vi "Server Sim.vi"() -> ()   [LabVIEW 2015]
uses:
  Type/TCP Packet Info.ctl
  Type/_RT Command.ctl
panel:
  in  "Stop Button":bool
  out "State":i32
  out "Response":string
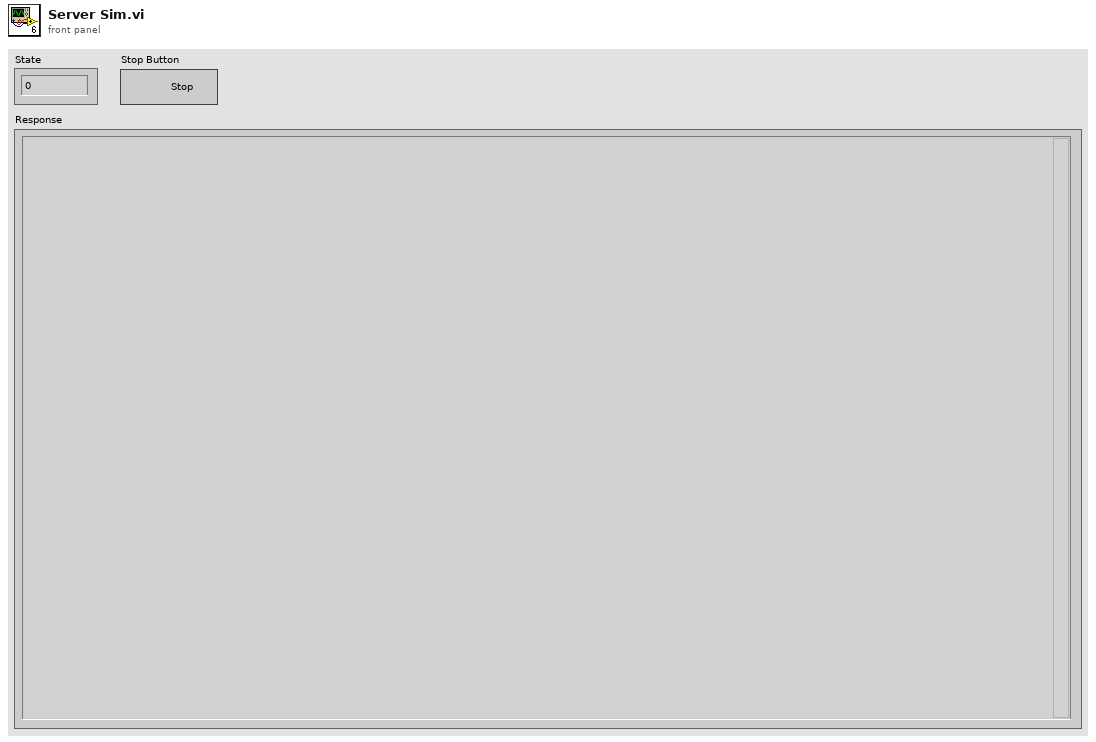
[diagram p1: front panel]
types:
  T1 = typedef "_RT Command.ctl" = enum16{"xml Start Run", "xml Start Actual Run", "xml Stop Run", "xml Runtime Update", "xml Get Status", "xml Get Table", "xml Set Table", "xml Get Configuration", "xml System Status", "xml Set LC Input Logic", "xml Get Data", "xml Get Info", "Start", "StartActualRun", "Stop", "Runtime Update", "Get Data", "Get Info", "Get Status", "Get Param", "Get Config", "Get Table", "Read ADC", "Set Oscillator", "Update Config", "Update Table", "Set All Pol", "Set Pol and DC", "Set Max Mass", "Toggle RP", "Toggle EL", "Set PIC", "Initialize Turbo", "Send Turbo Comm", "Close Turbo", "P1", "P2", "P3", "Send Serial", "Set LC Out", "Get LC In", "Read VAC", "Test Table", "Toggle Power", "Get Startup", "Set Startup", "Get ADC Table", "Set ADC Table", "Get Brief Status", "Get Detail Status", "Auxiliary Update", "Set CC Logics", "Set CC Input Logics", "Ignore Error", "invalid"}
  T2 = typedef "TCP Packet Info.ctl" = cluster{"Packet Signature":string, "Sequence Number":i32, "Command":T1, "Data Message Size":u32, "Data Message Size":string, "Data Message":string, "Error Message Size":u32, "Error Message Size":string, "Error Message":string, "Checksum":u32, "Error Message":errorcluster, "Command ID":string}
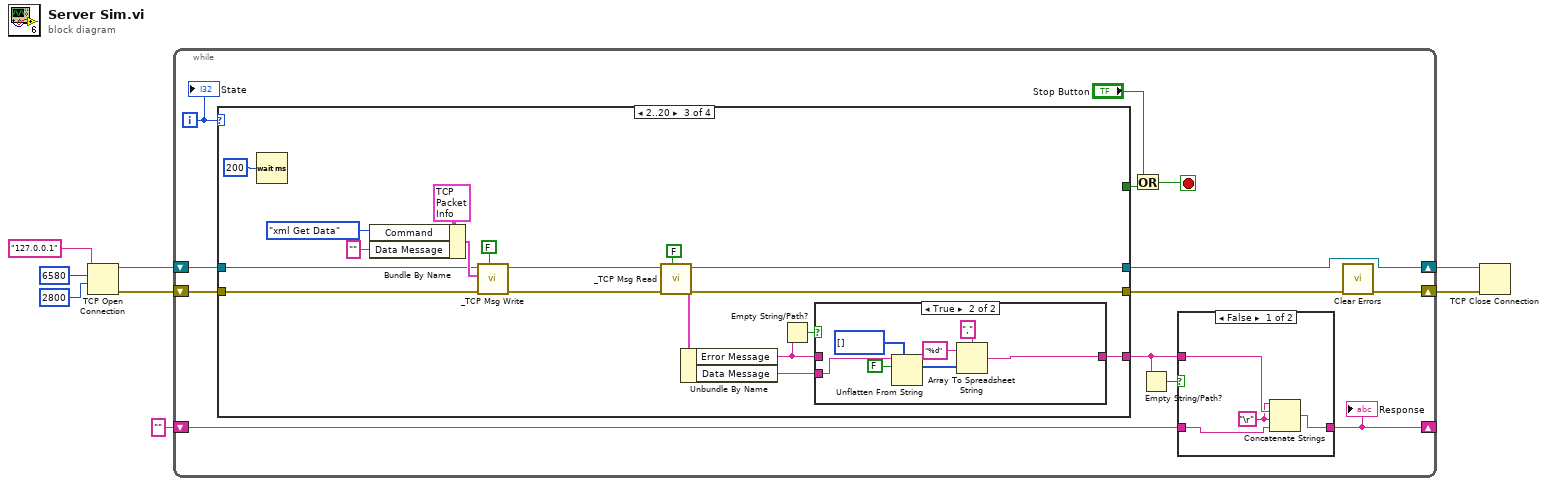
[diagram p0: block diagram]
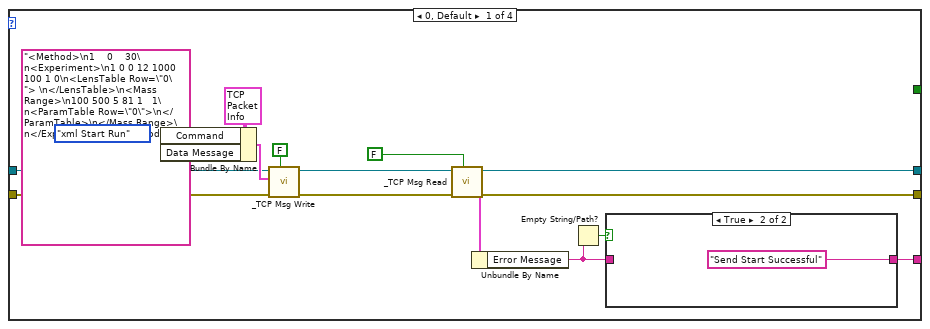
[diagram p3: hidden frame]
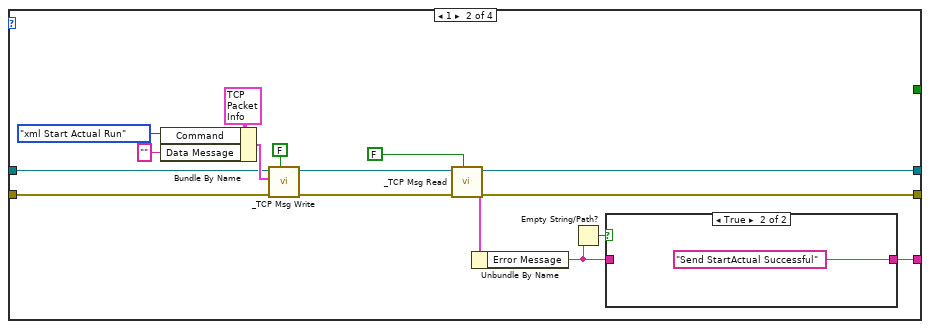
[diagram p5: hidden frame]
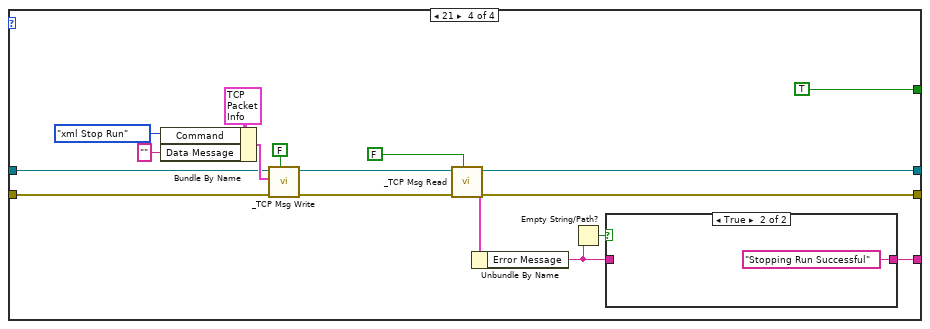
[diagram p8: hidden frame]
diagram:
  n1 = TCP Open Connection(address="127.0.0.1", remote port or service name=u16 6580 ("remote port"), timeout ms (60000)=2800) -> (connection ID=w5:refnum<k5>, error out=w4:errorcluster)  [unwired: 1 in, 1 out]
  n2 = while {
    shift-right: [w19] -> w3
    shift-left: w4 -> [w21]
    shift-right: [w16] -> w2
    shift-left: w5 -> [w20]
    shift-right: [w14] -> _
    shift-left: "" ("Data Message") -> [w15]
    i -> [w18]
    stop <- w10 stop-if-true
    n3 = case shown="2..20" w18 {
      tunnel: w21 -> [w38 w56 w76 w101]
      tunnel: w20 -> [w37 w55 w75 w100]
      tunnel: [w31 w49 w69 w94] -> w17
      tunnel: [w32 w50 w70 w95] -> w16
      tunnel: [w27 w45 w65 w90] -> w12
      tunnel: [_ _ _ TRUE] -> w13
      frame 0, Default {
        n4 = Bundle By Name(cluster=T2 {"Packet Signature"="", "Sequence Number"=0, "Command"=enum."Get Info", "Data Message Size"=0, "Data Message Size"="", "Data Message"="GI", "Error Message Size"=0, "Error Message Size"="", "Error Message"="", "Checksum"=0, "Error Message"={"status"=FALSE, "code"=0, "source"=""}, "Command ID"=""} ("Packet Info In"), "Command"=_RT_Command."xml Start Run", "Data Message"="<Method>\n1    0    30\n<Experiment>\n1 0 0 12 1000 100 1 0\n<LensTable Row=\"0\"> \n</LensTable>\n<Mass Range>\n100 500 5 81 1   1\n<ParamTable Row=\"0\">\n</ParamTable>\n</Mass Range>\n</Experiment>\n</Method>") -> (w41:T2)
        n5 = call "_TCP Msg Write.vi"("RT"=FALSE, "error in"=w38, "Packet Info In"=w41, "connection ID In"=w37) -> ("error out"=w34:errorcluster, "connection ID out"=w33:refnum<k5>)  [unwired: 1 in, 5 out]
        n6 = call "_TCP Msg Read.vi"("RT"=FALSE, "error in"=w34, "connection ID"=w33) -> ("error out"=w31:errorcluster, "Packet Info"=w30:T2, "connection ID out"=w32:refnum<k5>)  [unwired: 2 in, 4 out]
        n7 = Unbundle By Name(w30) -> ("Error Message"=w28:string)
        n8 = Empty String/Path?(string/path=w28) -> (empty?=w29:bool)
        n9 = case shown="True" w29 {
          tunnel: w28 -> [w43 _]
          tunnel: [w43 "Send Start Successful" ("Error Message")] -> w27
          frame False {
          }
          frame True {
          }
        }
      }
      frame 1 {
        n10 = Bundle By Name(cluster=T2 {"Packet Signature"="", "Sequence Number"=0, "Command"=enum."Get Info", "Data Message Size"=0, "Data Message Size"="", "Data Message"="GI", "Error Message Size"=0, "Error Message Size"="", "Error Message"="", "Checksum"=0, "Error Message"={"status"=FALSE, "code"=0, "source"=""}, "Command ID"=""} ("Packet Info In"), "Command"=_RT_Command."xml Start Actual Run", "Data Message"="") -> (w59:T2)
        n11 = call "_TCP Msg Write.vi"("RT"=FALSE, "error in"=w56, "Packet Info In"=w59, "connection ID In"=w55) -> ("error out"=w52:errorcluster, "connection ID out"=w51:refnum<k5>)  [unwired: 1 in, 5 out]
        n12 = call "_TCP Msg Read.vi"("RT"=FALSE, "error in"=w52, "connection ID"=w51) -> ("error out"=w49:errorcluster, "Packet Info"=w48:T2, "connection ID out"=w50:refnum<k5>)  [unwired: 2 in, 4 out]
        n13 = Unbundle By Name(w48) -> ("Error Message"=w46:string)
        n14 = Empty String/Path?(string/path=w46) -> (empty?=w47:bool)
        n15 = case shown="True" w47 {
          tunnel: w46 -> [w61 _]
          tunnel: [w61 "Send StartActual Successful" ("Error Message")] -> w45
          frame False {
          }
          frame True {
          }
        }
      }
      frame 2..20 {
        n16 = Wait (ms)(milliseconds to wait=u32 200) -> ()  [unwired: 1 out]
        n17 = Bundle By Name(cluster=T2 {"Packet Signature"="", "Sequence Number"=0, "Command"=enum."Get Info", "Data Message Size"=0, "Data Message Size"="", "Data Message"="GI", "Error Message Size"=0, "Error Message Size"="", "Error Message"="", "Checksum"=0, "Error Message"={"status"=FALSE, "code"=0, "source"=""}, "Command ID"=""} ("Packet Info In"), "Command"=_RT_Command."xml Get Data", "Data Message"="") -> (w79:T2)
        n18 = call "_TCP Msg Write.vi"("RT"=FALSE, "error in"=w76, "Packet Info In"=w79, "connection ID In"=w75) -> ("error out"=w72:errorcluster, "connection ID out"=w71:refnum<k5>)  [unwired: 1 in, 5 out]
        n19 = call "_TCP Msg Read.vi"("RT"=FALSE, "error in"=w72, "connection ID"=w71) -> ("error out"=w69:errorcluster, "Packet Info"=w68:T2, "connection ID out"=w70:refnum<k5>)  [unwired: 2 in, 4 out]
        n20 = Unbundle By Name(w68) -> ("Error Message"=w66:string, "Data Message"=w64:string)
        n21 = Empty String/Path?(string/path=w66) -> (empty?=w67:bool)
        n22 = case shown="True" w67 {
          tunnel: w66 -> [w81 _]
          tunnel: [w81 w83] -> w65
          tunnel: w64 -> [_ w88]
          frame False {
          }
          frame True {
            n23 = Unflatten From String(type=i32[] [], binary string=w88, data includes array or string size? (T)=FALSE) -> (value=w85:i32[])  [unwired: 2 in, 2 out]
            n24 = Array To Spreadsheet String(delimiter (Tab)=",", array=w85, 3:"%d" ("format string")) -> (spreadsheet string=w83:string)
          }
        }
      }
      frame 21 {
        n25 = Bundle By Name(cluster=T2 {"Packet Signature"="", "Sequence Number"=0, "Command"=enum."Get Info", "Data Message Size"=0, "Data Message Size"="", "Data Message"="GI", "Error Message Size"=0, "Error Message Size"="", "Error Message"="", "Checksum"=0, "Error Message"={"status"=FALSE, "code"=0, "source"=""}, "Command ID"=""} ("Packet Info In"), "Command"=_RT_Command."xml Stop Run", "Data Message"="") -> (w104:T2)
        n26 = call "_TCP Msg Write.vi"("RT"=FALSE, "error in"=w101, "Packet Info In"=w104, "connection ID In"=w100) -> ("error out"=w97:errorcluster, "connection ID out"=w96:refnum<k5>)  [unwired: 1 in, 5 out]
        n27 = call "_TCP Msg Read.vi"("RT"=FALSE, "error in"=w97, "connection ID"=w96) -> ("error out"=w94:errorcluster, "Packet Info"=w93:T2, "connection ID out"=w95:refnum<k5>)  [unwired: 2 in, 4 out]
        n28 = Unbundle By Name(w93) -> ("Error Message"=w91:string)
        n29 = Empty String/Path?(string/path=w91) -> (empty?=w92:bool)
        n30 = case shown="True" w92 {
          tunnel: w91 -> [w106 _]
          tunnel: [w106 "Stopping Run Successful" ("Error Message")] -> w90
          frame False {
          }
          frame True {
          }
        }
      }
    }
    n31 = Or(x="Stop Button", y=w13) -> (x .or. y?=w10:bool)
    n32 = Empty String/Path?(string/path=w12) -> (empty?=w11:bool)
    n33 = case shown="False" w11 {
      tunnel: w15 -> [w24 w26]
      tunnel: [w23 w26] -> w14
      tunnel: w12 -> [w25 _]
      frame False {
        w22 = "\r"
        n34 = Concatenate Strings(w22, w25, w22, w24) -> (w23:string)
      }
      frame True {
      }
    }
    "Response" <- w14
    n35 = call <vilib>:"Clear Errors.vi"("error in (no error)"=w17) -> ("error out"=w19:errorcluster)  [unwired: 5 in, 1 out]
    "State" <- w18
  }
  n36 = TCP Close Connection(connection ID=w2, error in (no error)=w3) -> ()  [unwired: 1 in, 2 out]
